vi "SW_Adjust_UI_draw_interwal.vi"(2 "UI update period (l.v.o.) in":i64, 3 "Historical CPU load, %":sgl) -> (0 "Updated?":bool, 1 "UI update period (l.v.o.) out":i64)   [LabVIEW 2018]
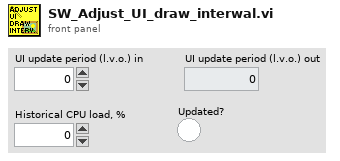
[diagram p1: front panel]
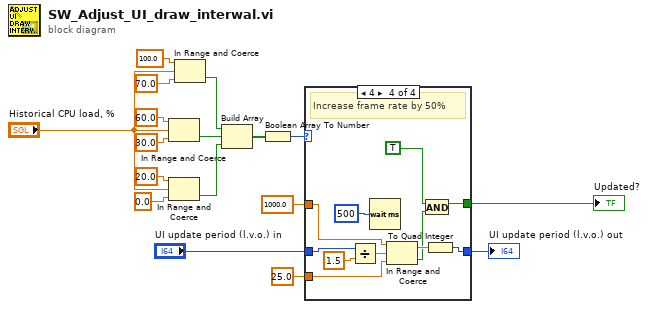
[diagram p0: block diagram]
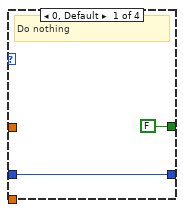
[diagram p2: hidden frame]
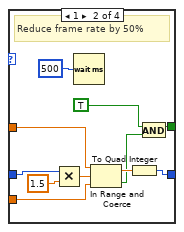
[diagram p3: hidden frame]
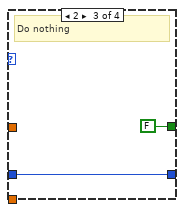
[diagram p4: hidden frame]
diagram:
  n1 = In Range and Coerce(upper limit=sgl 60.0, x="Historical CPU load, %", lower limit=sgl 30.0) -> (In Range?=w10:bool)  [unwired: 1 out]
  n2 = In Range and Coerce(upper limit=sgl 20.0, x="Historical CPU load, %", lower limit=sgl 0.0) -> (In Range?=w11:bool)  [unwired: 1 out]
  n3 = In Range and Coerce(upper limit=sgl 100.0, x="Historical CPU load, %", lower limit=sgl 70.0) -> (In Range?=w9:bool)  [unwired: 1 out]
  n4 = Build Array(w9, w10, w11) -> (w12:bool[])
  n5 = Boolean Array To Number(Boolean array=w12) -> (number=w13:u32)
  n6 = case shown="4" w13 {
    tunnel: "UI update period (l.v.o.) in" -> [w19 w30 w32 w43]
    tunnel: [w19 w26 w32 w38] -> w17
    tunnel: [FALSE w21 FALSE w34] -> w3
    tunnel: 1000.0 ("upper limit") -> [_ w23 _ w36]
    tunnel: 25.0 ("lower limit") -> [_ w25 _ w35]
    frame 0, Default {
      # "Do nothing"
    }
    frame 1 {
      # "Reduce frame rate by 50%"
      n7 = Multiply(x=w30, y=1.5) -> (x*y=w27:dbl)
      n8 = Wait (ms)(milliseconds to wait=u32 500) -> ()  [unwired: 1 out]
      n9 = In Range and Coerce(upper limit=w23, x=w27, lower limit=w25) -> (coerced(x)=w24:dbl, In Range?=w20:bool)
      n10 = To Quad Integer(1:w24) -> (0:w26:i64)
      n11 = And(x=TRUE, y=w20) -> (x .and. y?=w21:bool)
    }
    frame 2 {
      # "Do nothing"
    }
    frame 4 {
      # "Increase frame rate by 50%"
      n12 = Divide(x=w43, y=1.5) -> (x/y=w40:dbl)
      n13 = Wait (ms)(milliseconds to wait=u32 500) -> ()  [unwired: 1 out]
      n14 = In Range and Coerce(upper limit=w36, x=w40, lower limit=w35) -> (coerced(x)=w39:dbl, In Range?=w33:bool)
      n15 = And(x=TRUE, y=w33) -> (x .and. y?=w34:bool)
      n16 = To Quad Integer(1:w39) -> (0:w38:i64)
    }
  }
  "UI update period (l.v.o.) out" <- w17
  "Updated?" <- w3
